vi "Build Serial Cmd.vi"(6 "Display":string, 7 "Cmd":T1, 8 "error in (no error)":errorcluster, 9 "y":i64, 10 "x":i64, 11 "3022A in":refnum<class "3022A.lvclass">) -> (0 "error out":errorcluster, 2 "Cmd Out":string, 3 "3022A out":refnum<class "3022A.lvclass">)   [LabVIEW 2014, in "3022A.lvclass"]
uses:
  3022A.lvclass
  Controls/3022A/Ascii Cmd.ctl
  Controls/3022A/Enum Cmd.ctl
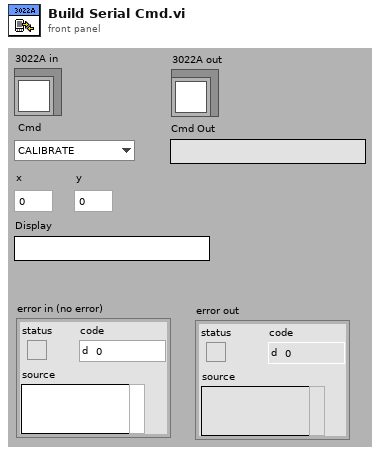
[diagram p1: front panel]
types:
  T1 = typedef "3022A.lvclass/Enum Cmd.ctl" = enum8{"CALIBRATE", "GET CAL DATA", "DUMP", "ESCAPE", "ID CAL LABEL", "INPUT CAL LABEL", "LIQUID LEVEL", "CONDENSER T", "SATURATOR T", "OPTICS T", "GET FLOW RATE", "READ ENV", "READ REF DETECTOR", "READ DETECTOR V", "READ 200 s BUFFER", "READ 20 s BUFFER", "READ 2 s BUFFER", "READ 1 s BUFFER", "READ PHOTOMETRIC CONC", "READ FP CONC", "READ MICROPROCESSOR PUMP CTL", "SENSOR", "SET VOLTAGE", "WRITE DISP MSG", "LASER OFF", "LASER ON", "PUMP OFF", "PUMP ON", "DRAIN", "FILL", "RESET CONC BUFFERS", "LOW FLOW MODE", "HIGH FLOW MODE"}
  T2 = typedef "3022A.lvclass/Ascii Cmd.ctl" = string[]
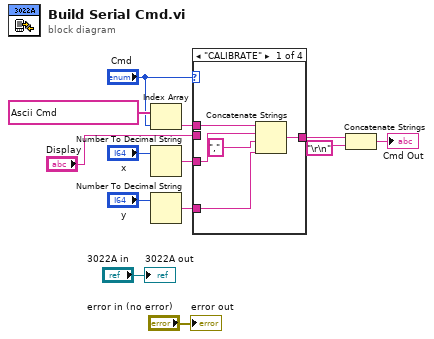
[diagram p0: block diagram]
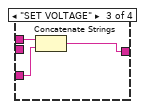
[diagram p3: hidden frame]
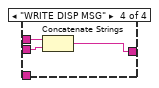
[diagram p4: hidden frame]
diagram:
  n1 = Index Array(array=T2 ["C", "C", "D", "ESC", "I", "L", "R0", "R1", "R2", "R3", "R4", "R5", "R6", "R7", "R8", "R9", "RA", "RB", "RC", "RD", "RE", "S", "V", "W", "X0", "X1", "X2", "X3", "X4", "X5", "X6", "X7", "X8"] ("RS232 CMD"), index="Cmd") -> (element=w11:string)
  n2 = Number To Decimal String(number="x") -> (decimal integer string=w6:string)  [unwired: 1 out]
  n3 = Number To Decimal String(number="y") -> (decimal integer string=w8:string)  [unwired: 1 out]
  n4 = case shown="\"CALIBRATE\"" "Cmd" {
    tunnel: w6 -> [w18 _ w21 _]
    tunnel: w8 -> [w16 _ _ _]
    tunnel: [w15 w19 w20 w24] -> w3
    tunnel: w11 -> [w14 w19 w22 w25]
    tunnel: "Display" -> [_ _ _ w23]
    frame "CALIBRATE" {
      n5 = Concatenate Strings(w14, w18, "," ("string"), w16) -> (w15:string)
    }
    frame "GET CAL DATA", Default {
    }
    frame "SET VOLTAGE" {
      n6 = Concatenate Strings(w22, w21) -> (w20:string)
    }
    frame "WRITE DISP MSG" {
      n7 = Concatenate Strings(w25, w23) -> (w24:string)
    }
  }
  n8 = Concatenate Strings(w3, "\r\n") -> (→"Cmd Out":string)
  "error out" <- "error in (no error)"
  "3022A out" <- "3022A in"
